vi "all-signals+drivingtorque-mean.vi"() -> ()   [LabVIEW 2018]
uses:
  <vilib>/Analysis/baseanly.llb/Mean (DBL).vi
  <vilib>/Analysis/NI_AALBase.lvlib
panel:
  out "RPM and dn":dynamicdata(graph)
  in  "stop driving torque":bool
  out "angular acc":dynamicdata(graph)
  in  "Clear Charts":bool
  in  "stop clear charts":bool
  in  "stop  counter (F)":bool caption="counter stop (F)"
  in  "stop I,U,M_brems (F)":bool caption="IU P STOP (F)"
  out "Driving Torque":dbl(graph)
  out "RPM":dbl
  in  "Messzeit in ms":u32=100 min=10 max=1000 step=10
  out "Bremsmoment":dynamicdata(graph)
  out "Strom, Spannung, elektrische Leistung":dynamicdata(graph)
  out "Geschwindigkeit":dynamicdata(graph)
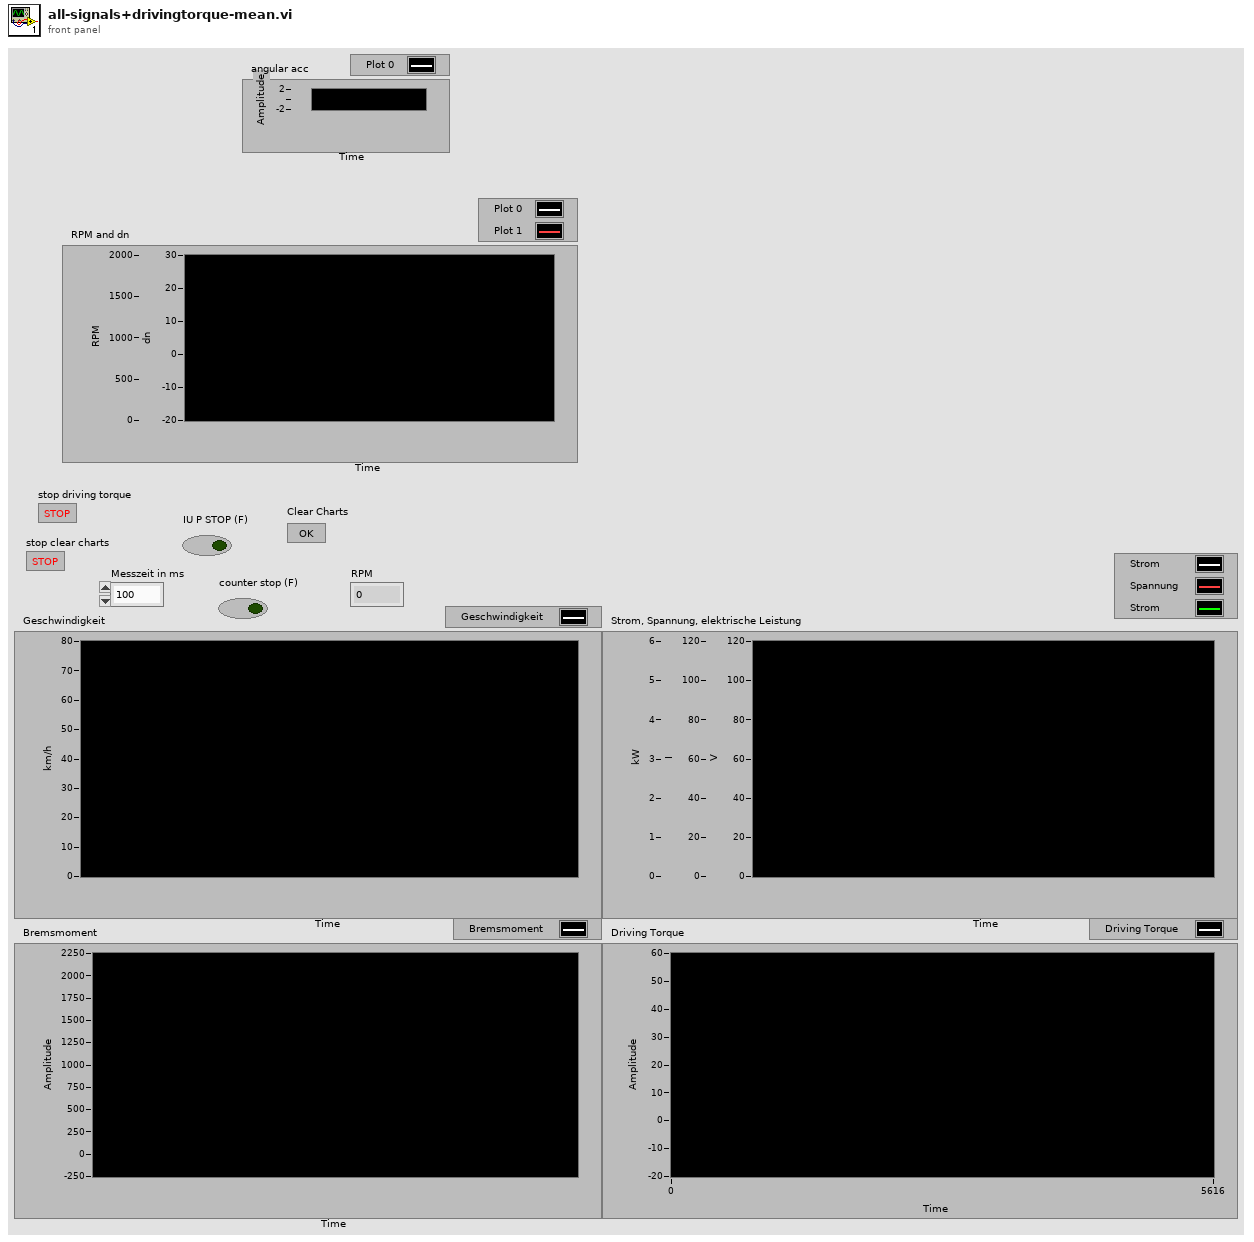
[diagram p1: front panel]
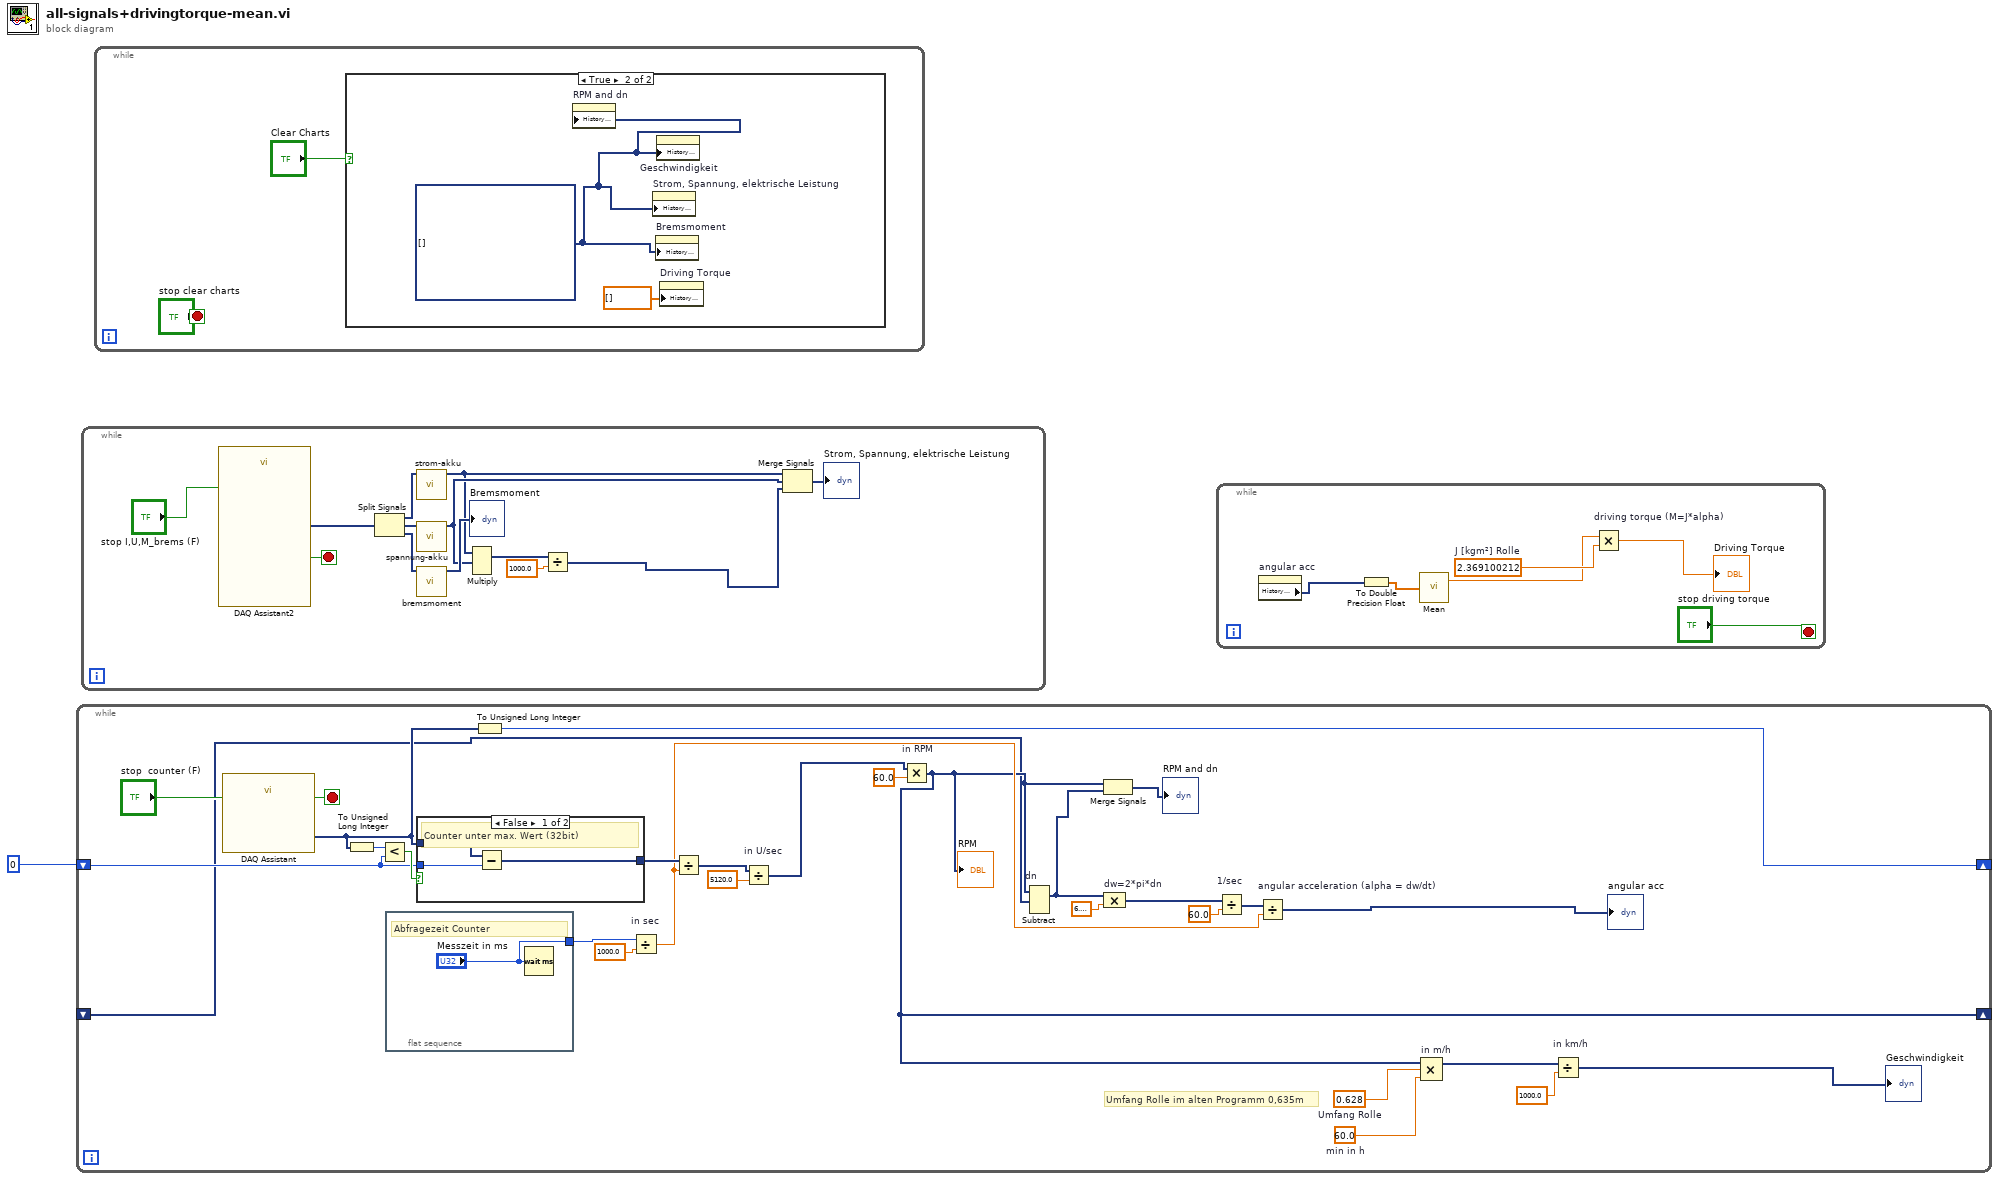
[diagram p0: block diagram]
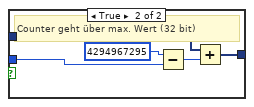
[diagram p2: hidden frame]
diagram:
  n1 = while {
    shift-right: [w28] -> _
    shift-left: u32 0 -> [w7]
    shift-right: [w6] -> _
    shift-left: _ -> [w4]
    stop <- w26 stop-if-true
    w13 = 60.0  # min in h
    w12 = 0.628  # Umfang Rolle
    # "Umfang Rolle im alten Programm 0,635m"
    n2 = call "DAQ Assistant"("stop (F)"="stop  counter (F)") -> ("data"=w8:dynamicdata, "stopped"=w26:bool)  [unwired: 15 in, 2 out]
    n3 = To Unsigned Long Integer(number=w8) -> (unsigned 32bit integer=w27:u32)
    n4 = Less?(x=w27, y=w7) -> (x < y?=w30:bool)
    n5 = flat-sequence {
      tunnel: ["Messzeit in ms"] -> w25
      frame #0 {
        # "Abfragezeit Counter"
        n6 = Wait (ms)(milliseconds to wait="Messzeit in ms") -> ()  [unwired: 1 out]
      }
    }
    n7 = case shown="False" w30 {
      tunnel: w8 -> [w34 w36]
      tunnel: w7 -> [w33 w38]
      tunnel: [w32 w35] -> w23
      frame False {
        # "Counter unter max. Wert (32bit)"
        n8 = Subtract(x=w34, y=w33) -> (x-y=w32:dynamicdata)
      }
      frame True {
        # "Counter geht über max. Wert (32 bit)"
        n9 = Subtract(x=u32 4294967295, y=w38) -> (x-y=w37:u32)
        n10 = Add(x=w36, y=w37) -> (x+y=w35:dynamicdata)
      }
    }
    n11 = To Unsigned Long Integer(number=w8) -> (unsigned 32bit integer=w28:u32)
    n12 = Divide "in sec"(x=w25, y=1000.0) -> (x/y=w16:dbl)
    n13 = Divide(x=w23, y=w16) -> (x/y=w22:dynamicdata)
    n14 = Divide "in U/sec"(x=w22, y=5120.0) -> (x/y=w10:dynamicdata)
    n15 = Multiply "in RPM"(x=w10, y=60.0) -> (x*y=w6:dynamicdata)
    "RPM" <- w6
    n16 = Subtract "dn"(1:w4, 2:w6) -> (0:w3:dynamicdata)  [unwired: 1 in, 1 out]
    n17 = Merge Signals(w6, w3) -> (→"RPM and dn":dynamicdata)
    n18 = Compound Arithmetic op=MULTIPLY "dw=2*pi*dn"(w3, 6.283185307179586) -> (w19:dynamicdata)
    n19 = Divide "1/sec"(x=w19, y=60.0) -> (x/y=w17:dynamicdata)
    n20 = Divide "angular acceleration (alpha = dw/dt)"(x=w17, y=w16) -> (x/y=→"angular acc":dynamicdata)
    n21 = Compound Arithmetic op=MULTIPLY "in m/h"(w6, w12, w13) -> (w14:dynamicdata)
    n22 = Divide "in km/h"(x=w14, y=1000.0) -> (x/y=→"Geschwindigkeit":dynamicdata)
  }
  n23 = while {
    stop <- w46 stop-if-true
    n24 = call "DAQ Assistant2"("stop (F)"="stop I,U,M_brems (F)") -> ("data"=w47:dynamicdata, "stopped"=w46:bool)  [unwired: 15 in, 2 out]
    n25 = Split Signals(w47) -> (w52:dynamicdata, w51:dynamicdata, w50:dynamicdata)  [unwired: 3 in]
    n26 = call "strom-akku.vi"("Dynamic Data"=w52) -> ("Filtered Signal"=w44:dynamicdata)  [unwired: 10 in]
    n27 = call "spannung-akku.vi"("Dynamic Data in"=w51) -> ("Dynamic Data out"=w45:dynamicdata)  [unwired: 10 in]
    n28 = call "bremsmoment.vi"("Dynamic Data in"=w50) -> ("Dynamic Data out"=→"Bremsmoment":dynamicdata)  [unwired: 10 in]
    n29 = Multiply(1:w45, 2:w44) -> (0:w42:dynamicdata)  [unwired: 1 in, 1 out]
    n30 = Divide(x=w42, y=1000.0) -> (x/y=w40:dynamicdata)
    n31 = Merge Signals(w44, w45, w40) -> (→"Strom, Spannung, elektrische Leistung":dynamicdata)
  }
  n32 = while {
    stop <- "stop clear charts" stop-if-true
    n33 = case shown="True" "Clear Charts" {
      frame False {
      }
      frame True {
        w55 = dynamicdata[] [] ("History Data")
        n34 = property on="RPM and dn" class="WFChart (strict)"("History Data"=w55) -> ()  [unwired: 2 in, 2 out]
        n35 = property on="Strom, Spannung, elektrische Leistung" class="WFChart (strict)"("History Data"=w55) -> ()  [unwired: 2 in, 2 out]
        n36 = property on="Bremsmoment" class="WFChart (strict)"("History Data"=w55) -> ()  [unwired: 2 in, 2 out]
        n37 = property on="Geschwindigkeit" class="WFChart (strict)"("History Data"=w55) -> ()  [unwired: 2 in, 2 out]
        n38 = property on="Driving Torque" class="WFChart (strict)"("History Data"=dbl[] []) -> ()  [unwired: 2 in, 2 out]
      }
    }
  }
  n39 = while {
    stop <- "stop driving torque" stop-if-true
    w61 = 2.369100212  # J [kgm²] Rolle
    n40 = property on="angular acc" class="WFChart (strict)"() -> ("History Data"=w57:dynamicdata[])  [unwired: 2 in, 2 out]
    n41 = To Double Precision Float(number=w57) -> (double precision float=w62:dbl[])
    n42 = call-poly <vilib>:"Mean.vi"("X"=w62) -> ("mean"=w59:dbl)  [unwired: 1 out]
    n43 = Multiply "driving torque (M=J*alpha)"(x=w59, y=w61) -> (x*y=→"Driving Torque":dbl)
  }
